vi "Valid Image.vi"(0 "image in":refnum<class "MSC Image.lvclass">, 5 "error in (no error)":errorcluster) -> (14 "image out":refnum<class "MSC Image.lvclass">, 15 "Valid Image?":bool, 19 "error out":errorcluster)   [LabVIEW 2014, in "MSC Image.lvclass"]
doc: "Checks if the image is valid. Use this function e.g. after pointer changing methods."
uses:
  MSC Image.lvclass
  controls/Size.ctl
  MSC Image.lvclass/MSC Image.ctl
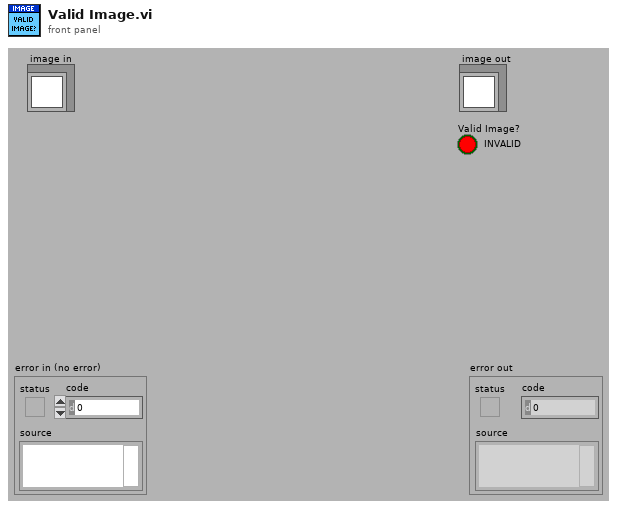
[diagram p1: front panel]
types:
  T1 = typedef "MSC Image.lvclass/Size.ctl" = cluster{"Cols":i32, "Rows":i32}
  T2 = typedef "Image.ctl" = cluster{"Pointer":u64, "Size":T3, "Image Type":T4, "Time Stamp":timestamp, "Variant":variant}
  T3 = typedef "Size.ctl" = cluster{"Cols":i32, "Rows":i32}
  T4 = typedef "Image Type.ctl" = i32
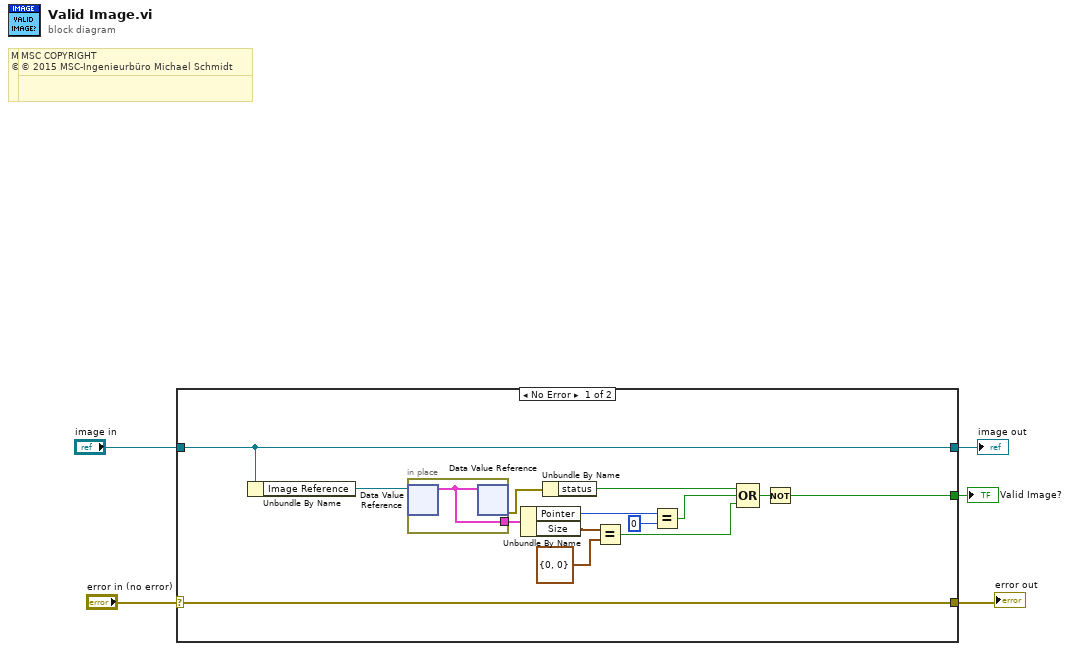
[diagram p0: block diagram]
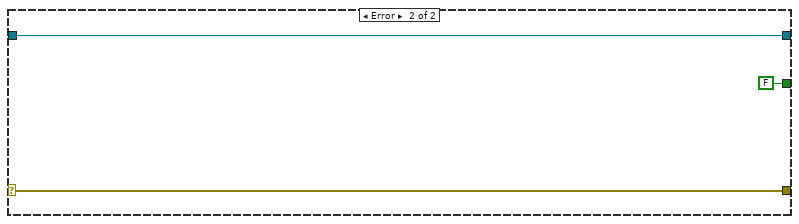
[diagram p2: hidden frame]
diagram:
  # "MSC COPYRIGHT\n© 2016 MSC-Ingenieurbüro Michael Schmidt"
  # "MSC COPYRIGHT\n© 2016 MSC-Ingenieurbüro Michael Schmidt"
  # "MSC COPYRIGHT\n© 2015 MSC-Ingenieurbüro Michael Schmidt"
  # "MSC COPYRIGHT\n© 2015 MSC-Ingenieurbüro Michael Schmidt"
  n1 = case shown="No Error" "error in (no error)" {
    selector: "error in (no error)" -> [w19 w23]
    tunnel: [w19 w23] -> w4
    tunnel: [w18 w22] -> w2
    tunnel: "image in" -> [w18 w22]
    tunnel: [w6 FALSE] -> w1
    frame No Error {
      n2 = Unbundle By Name(w18) -> ("Image Reference"=w17:refnum<data-value>)
      n3 = in-place {
        in-place-border: [w20] -> w16
        n4 = in-place-dvr #1(w17) -> (w20:T2)  [unwired: 1 out]
        n5 = in-place-dvr #1(w20) -> (w9:errorcluster)  [unwired: 1 out]
      }
      n6 = Unbundle By Name(w16) -> ("Pointer"=w15:u64, "Size"=w14:T3)
      n7 = Unbundle By Name(w9) -> ("status"=w8:bool)
      n8 = Equal?(x=w14, y=T1 {"Cols"=0, "Rows"=0} ("Size")) -> (x = y?=w10:bool)
      n9 = Equal?(x=w15, y=u64 0) -> (x = y?=w11:bool)
      n10 = Compound Arithmetic op=OR(w8, w11, w10) -> (w7:bool)
      n11 = Not(x=w7) -> (.not. x?=w6:bool)
    }
    frame Error {
    }
  }
  "error out" <- w4
  "image out" <- w2
  "Valid Image?" <- w1
